vi "Append Tabs To String Front.vi"(4 "TabCount(4)":i32=4, 5 "Str in":string="NEVSTOP-MemBuffer.lvlib:memBuffer.lvclass:replace memory subs") -> (2 "Str out":string="replace memory subs")   [LabVIEW 2014]
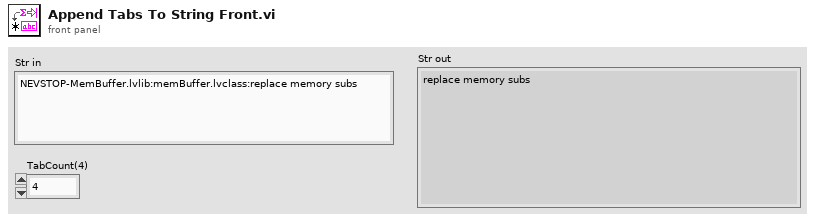
[diagram p1: front panel]
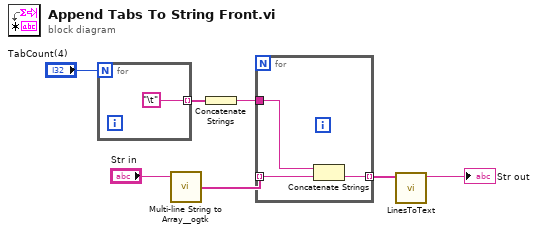
[diagram p0: block diagram]
diagram:
  n1 = for {
    N: "TabCount(4)" -> [_]
    tunnel: ["\t"] -> w2 mode=indexing
  }
  n2 = call <userlib>:"Multi-line String to Array__ogtk.vi"("string"="Str in") -> ("lines"=w4:string[])
  n3 = Concatenate Strings(w2) -> (w1:string)
  n4 = for {
    tunnel: [w10] -> w7 mode=indexing
    tunnel: w4 -> [w11] mode=indexing
    tunnel: w1 -> [w9]
    n5 = Concatenate Strings(w9, w11) -> (w10:string)
  }
  n6 = call "LinesToText.vi"("Lines"=w7) -> ("string"=→"Str out":string)  [unwired: 9 in, 1 out]
